vi "PROG 5 - Conversion of Temperatures Using Blocks.vi"() -> ()   [LabVIEW 2012]
panel:
  out "Numeric 2":dbl
  out "Numeric":dbl
  in  "Temperature (F)":dbl(slide) max=100.0 scale=0.0..100.0
  out "Thermometer (C)":dbl(slide) scale=0.0..100.0
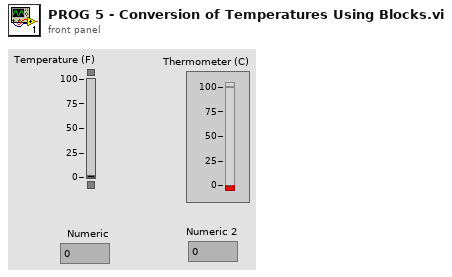
[diagram p1: front panel]
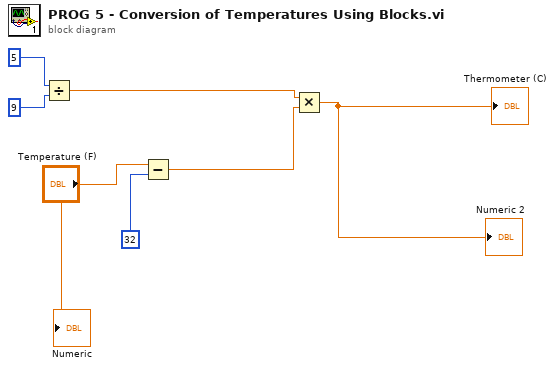
[diagram p0: block diagram]
diagram:
  n1 = Divide(x=5, y=9) -> (x/y=w3:dbl)
  n2 = Subtract(x="Temperature (F)", y=32) -> (x-y=w4:dbl)
  n3 = Multiply(x=w3, y=w4) -> (x*y=→"Thermometer (C)" →"Numeric 2":dbl)
  "Numeric" <- "Temperature (F)"
